vi "getStagesFromDB.vi"(8 "error in (no error)":errorcluster, 11 "ActionEditor in":refnum<class "ActionEditor.lvclass">) -> (0 "error out":errorcluster, 3 "ActionEditor out":refnum<class "ActionEditor.lvclass">)   [LabVIEW 2011, in "Views.lvlib" / "ScriptEditor.lvlib" / "ActionEditor.lvclass"]
uses:
  ActionEditor.lvclass
  ActionEditor.lvclass/ActionEditor.ctl
  Tools/DatabaseHelpers/DbConnection/DeviceDataBase/deviceDataBase.lvclass
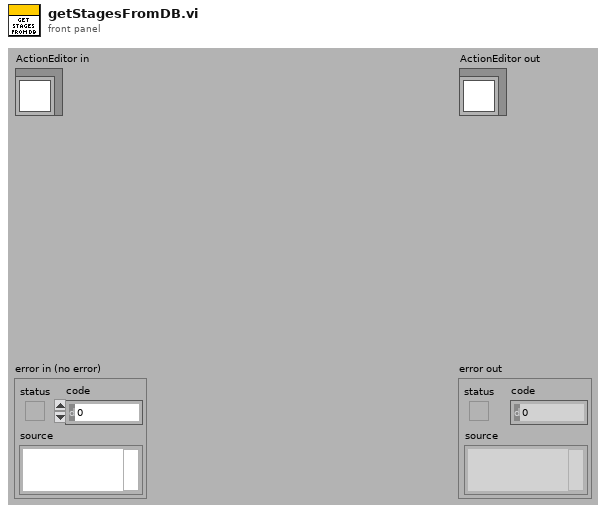
[diagram p1: front panel]
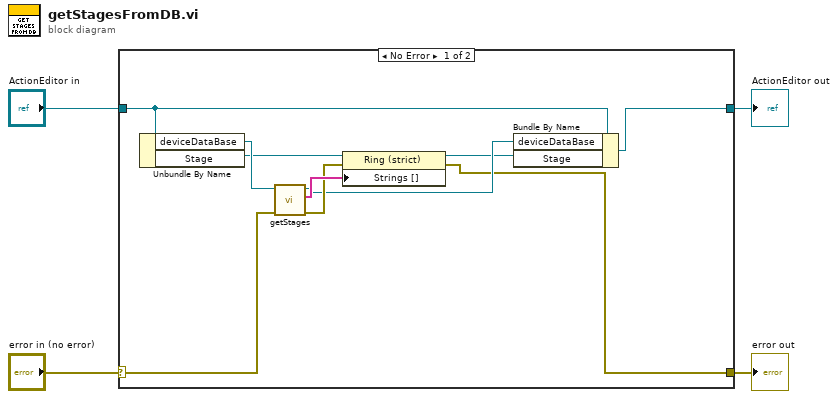
[diagram p0: block diagram]
diagram:
  n1 = case shown="No Error" "error in (no error)" {
    selector: "error in (no error)" -> [w5 w16]
    tunnel: [w6 w16] -> w3
    tunnel: [w7 w15] -> w1
    tunnel: "ActionEditor in" -> [w8 w15]
    frame No Error {
      n2 = Unbundle By Name(w8) -> ("deviceDataBase"=w14:refnum<class "deviceDataBase.lvclass">, "Stage"=w13:refnum<vi>)
      n3 = call "getStages.vi"("error in (no error)"=w5, "deviceDataBase in"=w14) -> ("error out"=w11:errorcluster, "stages"=w12:string[], "deviceDataBase out"=w10:refnum<class "deviceDataBase.lvclass">)  [unwired: 6 in, 1 out]
      n4 = property class="Ring (strict)"(reference=w13, error in=w11, "Strings []"=w12) -> (reference out=w9:refnum<vi>, error out=w6:errorcluster)
      n5 = Bundle By Name(cluster=w8, "deviceDataBase"=w10, "Stage"=w9) -> (w7:refnum<class "ActionEditor.lvclass">)
    }
    frame Error {
    }
  }
  "error out" <- w3
  "ActionEditor out" <- w1
